vi "Get camera angle and scale factor from trav moves.vi"(2 "dy (pix)":dbl, 3 "dx (pix)":dbl, 4 "dy (mm)":dbl, 5 "dx (mm)":dbl) -> (0 "scale factor (mm / pixel)":dbl, 1 "camera angle, ccw+ rel. to trav. (deg)":dbl)   [LabVIEW 2014]
uses:
  <vilib>/Analysis/baseanly.llb/Real Dot Product.vi
  <vilib>/Analysis/baseanly.llb/Unit Vector (DBL).vi
  <vilib>/Analysis/NI_AALBase.lvlib
  <vilib>/Analysis/NI_AALPro.lvlib
panel:
  # "Paul Nathan 11/06/2015"
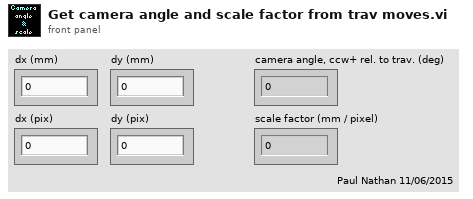
[diagram p1: front panel]
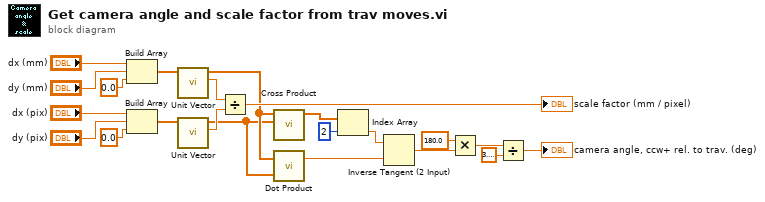
[diagram p0: block diagram]
diagram:
  n1 = Build Array("dx (mm)", "dy (mm)", 0.0 ("element")) -> (w16:dbl[])
  n2 = Build Array("dx (pix)", "dy (pix)", 0.0 ("element")) -> (w15:dbl[])
  n3 = call-poly <vilib>:"Unit Vector.vi"("Input Vector"=w16) -> ("norm"=w14:dbl, "Unit Vector"=w11:dbl[])  [unwired: 8 in, 1 out]
  n4 = call-poly <vilib>:"Unit Vector.vi"("Input Vector"=w15) -> ("norm"=w13:dbl, "Unit Vector"=w10:dbl[])  [unwired: 8 in, 1 out]
  n5 = Divide(x=w14, y=w13) -> (x/y=→"scale factor (mm / pixel)":dbl)
  n6 = call <vilib>:"Cross Product.vi"("B Vector"=w10, "A Vector"=w11) -> ("Cross Product"=w9:dbl[])  [unwired: 8 in, 1 out]
  n7 = call-poly <vilib>:"Dot Product.vi"("Y Vector"=w10, "X Vector"=w11) -> ("X * Y"=w6:dbl)  [unwired: 1 out]
  n8 = Index Array(array=w9, index=2) -> (element=w7:dbl)
  n9 = Inverse Tangent (2 Input)(1:w6, 2:w7) -> (0:w5:dbl)
  n10 = Multiply(x=180.0 ("y"), y=w5) -> (x*y=w4:dbl)
  n11 = Divide(x=w4, y=3.141592653589793) -> (x/y=→"camera angle, ccw+ rel. to trav. (deg)":dbl)
